vi "PH_SSAC.PC Write PSDB.vi"(0 "i ref in":refnum<vi>, 5 "error IO":errorcluster) -> (14 "i ref out":refnum<vi>, 19 "error out":errorcluster)   [LabVIEW 2014, in "PH_SSAC.lvlib"]
doc: "This is the proc case which sets the data to be written to the to the PHELIX shot data base."
uses:
  PH_SSAC.lvlib
  PH_PSDBWriter/PH_PSDBWriter.2D dataset.ctl
  User/Eisenbarth/psdb_lv/PSDB_AxisDescription.ctl
  PH_Common/PH_Common.lvlib
  PH_PSDBWriter/PH_PSDBWriter.lvlib
  PH_StatusHandler/PH_StatusHandler.lvlib
  User/Eisenbarth/psdb_lv/PSDB.lvlib
panel:
  in  "2D data":T1
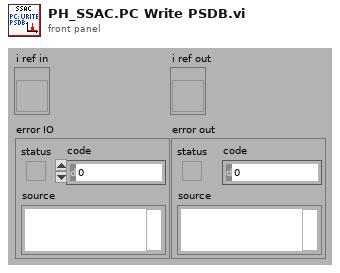
[diagram p1: front panel]
types:
  T1 = typedef "PH_PSDBWriter.lvlib/PH_PSDBWriter.2D dataset.ctl" = cluster{"name":string, "data":dbl[][], "axis description":T2}
  T2 = typedef "PSDB.lvlib/PSDB_AxisDescription.ctl" = cluster{"x axis label":string, "y axis label":string, "x axis unit":string, "y axis unit":string}
  T3 = typedef "PH_StatusHandler.lvlib/PH_StatusHandler.Status.ctl" = i16
  T4 = typedef "PH_SSAC.lvlib/PH_SSAC.i attribute.ctl" = cluster{"GUI Refs":cluster{"Delete":refnum<vi>, "Global On":refnum<vi>, "Cam Source":refnum<vi>, "Frame Main Signal":refnum<vi>, "Frame Background":refnum<vi>, "dt (Gauss smooth)":refnum<vi>, "Calibration Factor":refnum<vi>, "Background acquire":refnum<vi>, "Threshold":refnum<vi>, "Time evolution of mean pulse duration":refnum<vi>, "Mean Pulse Duration":refnum<vi>, "Main signal":refnum<vi>, "Current Pulse Duration":refnum<vi>, "Processed":refnum<vi>, "Saturation":refnum<vi>, "# for Average":refnum<vi>, "Position":refnum<vi>, "BG Status":refnum<vi>, "Save BG data":refnum<vi>, "Read BG Data":refnum<vi>, "Background Calibration Data":refnum<vi>}, "Images":cluster{"OP Image":T5, "GUI Image":T5, "PSDB Image":T5}, "Global On?":bool, "Frame Main":cluster{"x":u32, "dx":u32, "y":u32, "dy":u32}, "Frame Background":cluster{"x":u32, "dx":u32, "y":u32, "dy":u32}, "dt [fs]":dbl, "Calibration Factor [fs/pixel]":dbl, "Threshold":dbl, "Time evolution of mean pulse duration [fs]":dbl[], "Main Signal":cluster{"Time for Main":dbl[], "Signal":dbl[]}, "Processed":bool, "Current Pulse Duration [fs]":dbl, "# for Average":i32, "Position":i32, "Pulse Durations [fs]":dbl[], "BG":cluster{"Acquire?":bool, "Background Calibration Data":T6, "Save Data":bool}}
  T5 = typedef "IMAQ Image.ctl" = refnum<image>
  T6 = typedef "PH_SSAC.lvlib/PH_SSAC.Background Data.ctl" = cluster{"Date":string, "Time":string, "Frame Main":cluster{"x":u32, "dx":u32, "y":u32, "dy":u32}, "dt [fs]":dbl, "Calibration Factor [fs/pixel]":dbl, "Signal":dbl[], "Frame Background":cluster{"x":u32, "dx":u32, "y":u32, "dy":u32}}
  T7 = typedef "PH_PSDBWriter.lvlib/PH_PSDBWriter.Boolean dataset.ctl" = cluster{"name":string, "data":bool, "unit":string}
  T8 = typedef "PH_PSDBWriter.lvlib/PH_PSDBWriter.Image dataset.ctl" = cluster{"name":string, "data":T5, "unit":string}
  T9 = typedef "PH_PSDBWriter.lvlib/PH_PSDBWriter.Numeric dataset.ctl" = cluster{"name":string, "data":dbl, "unit":string}
  T10 = typedef "PH_PSDBWriter.lvlib/PH_PSDBWriter.String dataset.ctl" = cluster{"name":string, "data":string, "unit":string}
  T11 = typedef "PH_PSDBWriter.lvlib/PH_PSDBWriter.PSDB Dataset.ctl" = cluster{"Version":i32, "2D data Input":T1[], "Boolean Input":T7[], "Image Input":T8[], "Numeric Input":T9[], "String Input":T10[]}
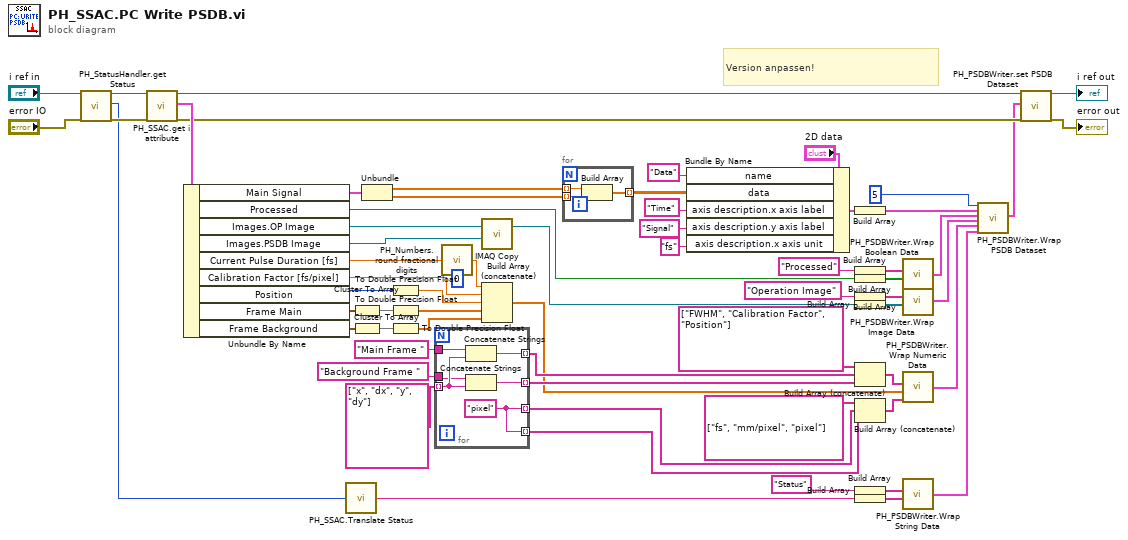
[diagram p0: block diagram]
diagram:
  # "Version anpassen!"
  n1 = call "PH_StatusHandler.get Status.vi"("VI in"="i ref in", "error in"="error IO") -> ("VI out"=w2:refnum<vi>, "Status"=w1:T3, "error out"=w4:errorcluster)  [unwired: 15 in]
  n2 = call "PH_SSAC.get i attribute.vi"("i ref in"=w2, "error in (no error)"=w4) -> ("i ref out"=w30:refnum<vi>, "i attribute"=w64:T4, "error out"=w63:errorcluster)  [unwired: 15 in]
  n3 = Unbundle By Name(w64) -> ("Main Signal"=w60:cluster{"Time for Main":dbl[], "Signal":dbl[]}, "Processed"=w13:bool, "Images.OP Image"=w6:T5, "Images.PSDB Image"=w5:T5, "Current Pulse Duration [fs]"=w40:dbl, "Calibration Factor [fs/pixel]"=w32:dbl, "Position"=w55:i32, "Frame Main"=w53:cluster{"x":u32, "dx":u32, "y":u32, "dy":u32}, "Frame Background"=w52:cluster{"x":u32, "dx":u32, "y":u32, "dy":u32})
  n4 = call "PH_SSAC.Translate Status.vi"("Device Status"=w1) -> ("Translated Status"=w23:string)
  n5 = Cluster To Array(cluster=w53) -> (array=w51:u32[])
  n6 = Cluster To Array(cluster=w52) -> (array=w50:u32[])
  n7 = Unbundle(w60) -> ("Time for Main"=w59:dbl[], "Signal"=w58:dbl[])
  n8 = To Double Precision Float(number=w55) -> (double precision float=w54:dbl)
  n9 = To Double Precision Float(number=w51) -> (double precision float=w49:dbl[])
  n10 = To Double Precision Float(number=w50) -> (double precision float=w48:dbl[])
  n11 = for {
    tunnel: string[] ["x", "dx", "y", "dy"] -> [w70] mode=indexing
    tunnel: "Main Frame " -> [w71]
    tunnel: "Background Frame " -> [w69]
    tunnel: [w68] -> w43 mode=indexing
    tunnel: [w67] -> w44 mode=indexing
    tunnel: [w66] -> w42 mode=indexing
    tunnel: [w66] -> w41 mode=indexing
    w66 = "pixel"
    n12 = Concatenate Strings(w71, w70) -> (w67:string)
    n13 = Concatenate Strings(w69, w70) -> (w68:string)
  }
  n14 = call "PH_Numbers.round fractional digits.vi"("Input"=w40, "Position (1)"=i16 0) -> ("round Output"=w39:dbl)
  n15 = call "IMAQ Copy"("Image Dst"=w5, "Image Src"=w6) -> ("Image Dst Out"=w7:T5)  [unwired: 4 in, 1 out]
  n16 = Build Array (concatenate)(w39, w32, w54, w49, w48) -> (w18:dbl[])
  n17 = for {
    tunnel: w59 -> [w74] mode=indexing
    tunnel: w58 -> [w73] mode=indexing
    tunnel: [w72] -> w34 mode=indexing
    n18 = Build Array(w74, w73) -> (w72:dbl[])
  }
  n19 = Bundle By Name(cluster="2D data", "name"="Data", "data"=w34, "axis description.x axis label"="Time", "axis description.y axis label"="Signal", "axis description.x axis unit"="fs") -> (w61:T1)
  n20 = Build Array(w61) -> (w8:T1[])
  n21 = Build Array("Processed") -> (w11:string[])
  n22 = Build Array(w13) -> (w10:bool[])
  n23 = Build Array("Operation Image") -> (w15:string[])
  n24 = Build Array(w7) -> (w14:T5[])
  n25 = Build Array (concatenate)(string[] ["FWHM", "Calibration Factor", "Position"], w44, w43) -> (w17:string[])
  n26 = Build Array (concatenate)(string[] ["fs", "mm/pixel", "pixel"], w42, w41) -> (w19:string[])
  n27 = Build Array("Status" ("name")) -> (w21:string[])
  n28 = Build Array(w23) -> (w20:string[])
  n29 = call "PH_PSDBWriter.Wrap Boolean Data.vi"("Data Array"=w10, "Name Array"=w11) -> ("PSDB Boolean Data Array"=w25:T7[])  [unwired: 2 in]
  n30 = call "PH_PSDBWriter.Wrap Image Data.vi"("Data Arrray"=w14, "Name Array"=w15) -> ("PSDB Image Data Array"=w26:T8[])  [unwired: 2 in]
  n31 = call "PH_PSDBWriter.Wrap Numeric Data.vi"("Unit Array"=w19, "Data Array"=w18, "Name Array"=w17) -> ("PSDB Numeric Data Array"=w27:T9[])  [unwired: 1 in]
  n32 = call "PH_PSDBWriter.Wrap String Data.vi"("Data Array"=w20, "Name Array"=w21) -> ("PSDB String Data Array"=w28:T10[])  [unwired: 2 in]
  n33 = call "PH_PSDBWriter.Wrap PSDB Dataset.vi"("Version"=5, "2D data Input"=w8, "Boolean Input"=w25, "Image Input"=w26, "Numeric Input"=w27, "String Input"=w28) -> ("PSDB Dataset"=w24:T11)  [unwired: 13 in]
  n34 = call "PH_PSDBWriter.set PSDB Dataset.vi"("VI in"=w30, "PSDB Dataset"=w24, "error in (no error)"=w63) -> ("VI out"=→"i ref out":refnum<vi>, "error out"=→"error out":errorcluster)  [unwired: 15 in]
